vi "TestLocalize2.vi"() -> ()   [LabVIEW 2011]
uses:
  JelmersTracker.llb/TrackerDLL.vi
panel:
  out "debug output":T1(plugin-control)
  out "max Y pos":i32
  out "max X pos":i32
  out "X profile":sgl[](graph)
  out "Y profile":sgl[](graph)
  out "Y autocor":sgl[](graph)
  out "X autocor":sgl[](graph)
  out "xcor position":cluster{"X":sgl, "Y":sgl}
  in  "y":sgl
  in  "x":sgl
  out "COM position":cluster{"X":sgl, "Y":sgl}
  in  "iterations":i32=2
  out "median":sgl
  in  "Path":path
  in  "Browse?":bool
  out "Radial profile":sgl[](graph)
  in  "debug library":bool
  out "Image":T1(plugin-control)
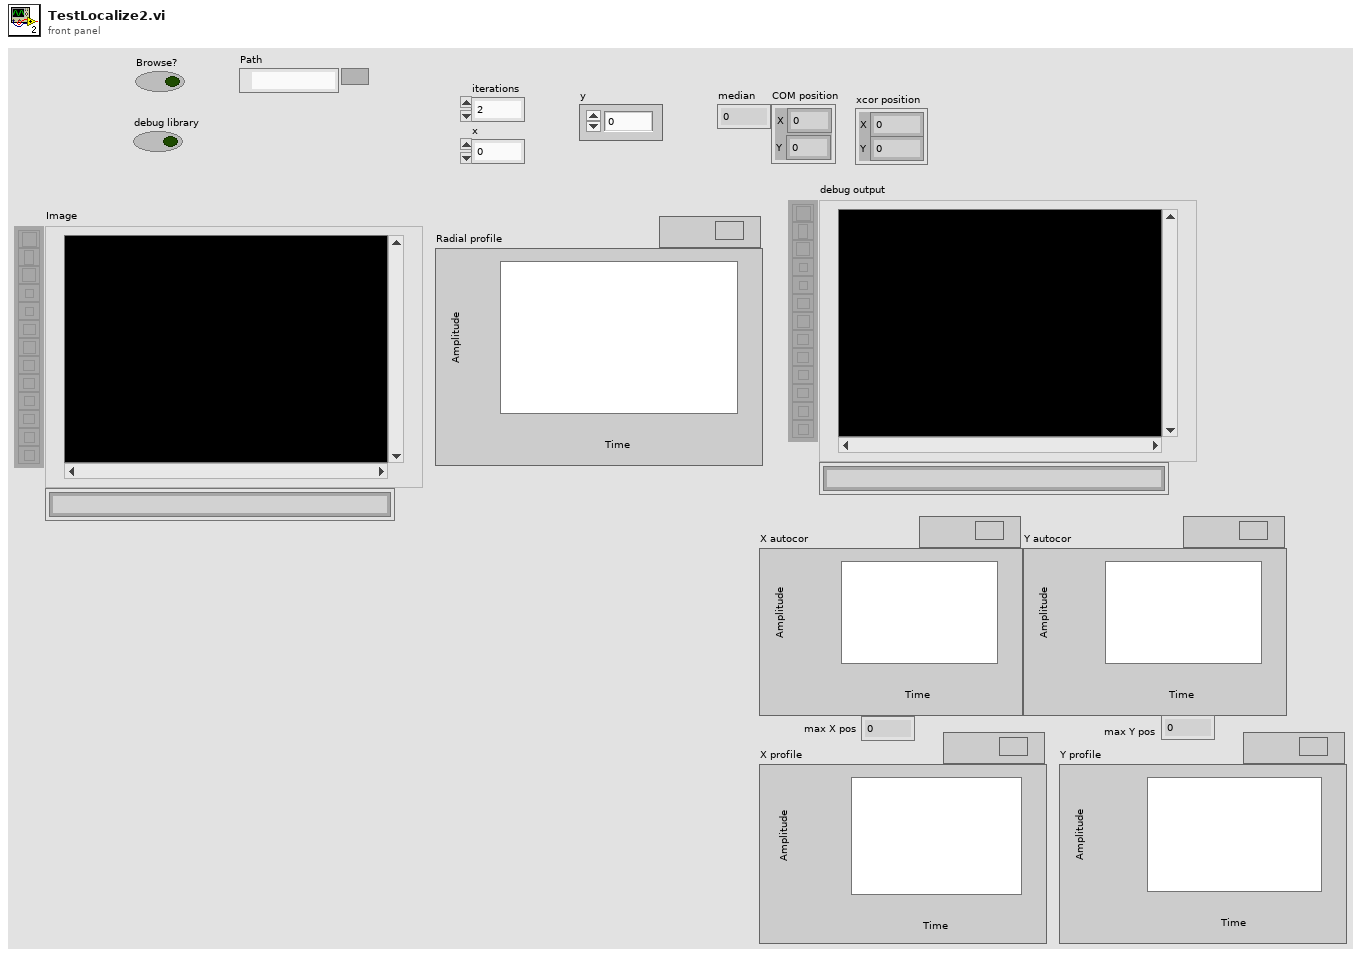
[diagram p1: front panel]
types:
  T1 = typedef "IMAQ Image.ctl" = refnum<image>
  T2 = typedef "Image Type" = u32
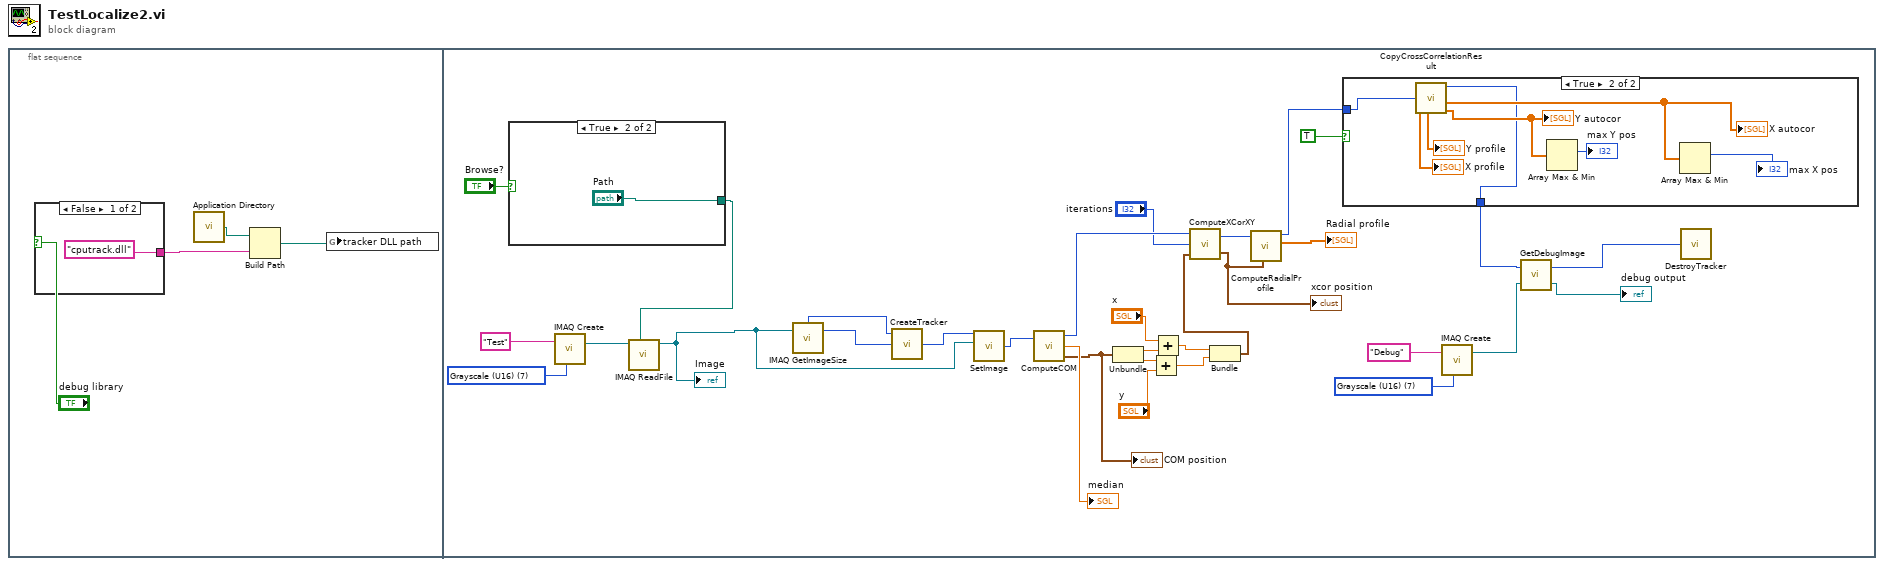
[diagram p0: block diagram]
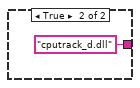
[diagram p2: hidden frame]
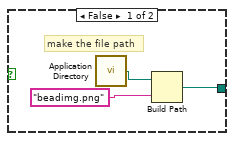
[diagram p3: hidden frame]
diagram:
  n1 = flat-sequence {
    frame #0 {
      n2 = case shown="False" "debug library" {
        tunnel: ["cputrack.dll" "cputrack_d.dll"] -> w3
        frame False {
        }
        frame True {
        }
      }
      n3 = call <vilib>:"Application Directory.vi"() -> ("Application Directory"=w2:path)
      n4 = Build Path(base path=w2, name or relative path=w3) -> (appended path=w4:path)
      n5 = global write "TrackerDLL.vi" "tracker DLL path"(w4) -> ()
    }
    frame #1 {
      w33 = T2 7 items=["Grayscale (U8)", "Grayscale (I16)", "Grayscale (SGL)", "Complex (CSG)", "RGB (U32)", "HSL (U32)", "RGB (U64)", "Grayscale (U16)"] ("Image Type")
      w35 = T2 7 items=["Grayscale (U8)", "Grayscale (I16)", "Grayscale (SGL)", "Complex (CSG)", "RGB (U32)", "HSL (U32)", "RGB (U64)", "Grayscale (U16)"] ("Image Type")
      n6 = case shown="True" "Browse?" {
        tunnel: [w39 "Path"] -> w36
        frame False {
          # "make the file path"
          n7 = call <vilib>:"Application Directory.vi"() -> ("Application Directory"=w40:path)
          n8 = Build Path(base path=w40, name or relative path="beadimg.png") -> (appended path=w39:path)
        }
        frame True {
        }
      }
      n9 = call "IMAQ Create"("Image Name"="Test" ("String"), "Image Type"=w35) -> ("New Image"=w37:T1)  [unwired: 3 in, 1 out]
      n10 = call "IMAQ ReadFile"("File Path"=w36, "Image"=w37) -> ("Image Out"=w25:T1)  [unwired: 5 in, 4 out]
      "Image" <- w25
      n11 = call "IMAQ GetImageSize"("Image"=w25) -> ("Y Resolution"=w31:i32, "X Resolution"=w32:i32)  [unwired: 3 in, 1 out]
      n12 = call "CreateTracker.vi"("height"=w31, "width"=w32) -> ("return type"=w26:u64)  [unwired: 1 in]
      n13 = call "SetImage.vi"("Image"=w25, "tracker"=w26) -> ("tracker"=w24:u64)  [unwired: 2 in]
      n14 = call "ComputeCOM.vi"("tracker"=w24) -> ("tracker"=w23:u64, "median"=→"median":sgl, "position"=w18:cluster{"X":sgl, "Y":sgl})  [unwired: 1 in]
      "COM position" <- w18
      n15 = Unbundle(w18) -> ("X"=w17:sgl, "Y"=w14:sgl)
      n16 = Add(x=w14, y="y") -> (x+y=w13:sgl)
      n17 = Add(x="x", y=w17) -> (x+y=w15:sgl)
      n18 = Bundle(w15, w13) -> (w11:cluster{sgl, sgl})  [unwired: 1 in]
      n19 = call "ComputeXCorXY.vi"("position"=w11, "iterations"="iterations", "tracker"=w23) -> ("position"=w19:cluster{"X":sgl, "Y":sgl}, "tracker"=w20:u64)
      "xcor position" <- w19
      n20 = call "ComputeRadialProfile.vi"("center"=w19, "tracker"=w20) -> ("output"=→"Radial profile":sgl[], "tracker"=w29:u64)  [unwired: 8 in]
      n21 = case shown="True" TRUE {
        tunnel: w29 -> [w43 w45]
        tunnel: [w43 w44] -> w10
        frame False {
        }
        frame True {
          n22 = call "CopyCrossCorrelationResult.vi"("tracker"=w45) -> ("x prof"=→"X profile":sgl[], "y prof"=→"Y profile":sgl[], "tracker"=w44:u64, "x result"=w49:sgl[], "y_result"=w48:sgl[])  [unwired: 3 in]
          "X autocor" <- w49
          "Y autocor" <- w48
          n23 = Array Max & Min(array=w48) -> (max index (indices)=→"max Y pos":i32)  [unwired: 3 out]
          n24 = Array Max & Min(array=w49) -> (max index (indices)=→"max X pos":i32)  [unwired: 3 out]
        }
      }
      n25 = call "IMAQ Create"("Image Name"="Debug" ("String"), "Image Type"=w33) -> ("New Image"=w8:T1)  [unwired: 3 in, 1 out]
      n26 = call "GetDebugImage.vi"("image"=w8, "tracker"=w10) -> ("image"=→"debug output":T1, "tracker"=w9:u64)
      n27 = call "DestroyTracker.vi"("tracker"=w9) -> ()
    }
  }
